vi "SMTP Email Not An SMTP Session_.vi"(1 "smtp session":T1) -> (0 "not an smtp session?":bool)   [LabVIEW 2009, in "NewNI_SMTPEmail.lvlib"]
uses:
  NewNI_SMTPEmail.lvlib
  SMTP Email Session.ctl
panel:
  in  "tcp connection":refnum<k5>
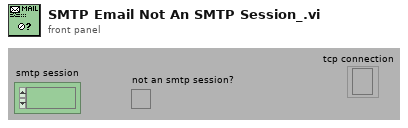
[diagram p1: front panel]
types:
  T1 = typedef "NewNI_SMTPEmail.lvlib/SMTP Email Session.ctl" = refnum<k1>
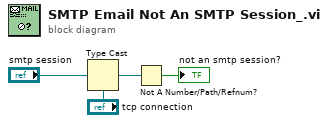
[diagram p0: block diagram]
diagram:
  n1 = Type Cast(type="tcp connection", x="smtp session") -> (*(type *) &x=w2:refnum<k5>)
  n2 = Not A Number/Path/Refnum?(number/path/refnum=w2) -> (NaN/Path/Refnum?=→"not an smtp session?":bool)
